vi "Main.Cleanup.vi"(11 "State Variables":T1={"Main App"={"Device Error"={"status"=FALSE, "code"=0, "source"=""}, "FPGA Session"=0, "Incoming Decimation"=0, "Outgoing Decimation"=0, "Process"=refnum}, "Protocol App"={"XNET Settings"={"Database"="", "Cluster"="", "Port"="", "Baud rate [Bd]"=0, "Termination"=0, "Incoming Rate"=0, "Outcoming Rate"=1, "Write Decimation"=1}, "Data"=[], "DTCs"=[], "Sim Addresses LUT"=variant, "Data Table LUT"=variant, "MonitorTool.Network"={"Address"=0, "Name"=0}, "Name"=""}} {"Protocol App"."MonitorTool.Network"."Name" format="%.0x"; "Protocol App"."Data"."Trigger.Refs"."Data Reference" format="%.0x"; "Protocol App"."Data"."Disable.Refs"."Data Reference" format="%.0x"; "Protocol App"."Data"."Timing.Refs"."Data Reference" format="%.0x"; "Protocol App"."Data"."Network"."Name" format="%.0x"; "Protocol App"."Data"."Incoming.Refs"."Data Reference" format="%.0x"; "Protocol App"."Data"."Outgoing.Refs"."Data Reference" format="%.0x"; "Protocol App"."XNET Settings"."Termination" items=["Off", "On"]}) -> (0 "error out":errorcluster)   [LabVIEW 2015, in "J1939 Addon Engine.lvlib"]
uses:
  J1939 Addon Engine.lvlib
  Types/Main.State Variables.ctl
  <vilib>/NI/NIVS Inline Async API/_VS Inline Async API/VS Inline Async API/VS Inline Async API.lvclass
  Types/Main.Settings.ctl
  Types/Protocol.App Settings.ctl
  Shared/Types/XNET Settings.ctl
  Types/Protocol.XNET Refs.ctl
  Shared/Types/Monitor Settings.ctl
  <vilib>/NI Veristand/Custom Device API/Block Data Reference.ctl
  <vilib>/NI Veristand/Custom Device API/Data Reference.ctl
  Types/Main.Outgoing.Frame.Settings.ctl
  Shared/Types/Outgoing Event Trigger Types.ctl
  Types/Engine.DTC Settings.ctl
  Shared/Types/Compiled Simulated Settings.ctl
  Types/Engine.DTC FIFOs.ctl
  <vilib>/xnet/xnet.llb/XNET Database Close (Database).vi
  <vilib>/NI VeriStand/Custom Device API/Custom Device API.lvlib
  Shared/J1939 Addon Shared.lvlib
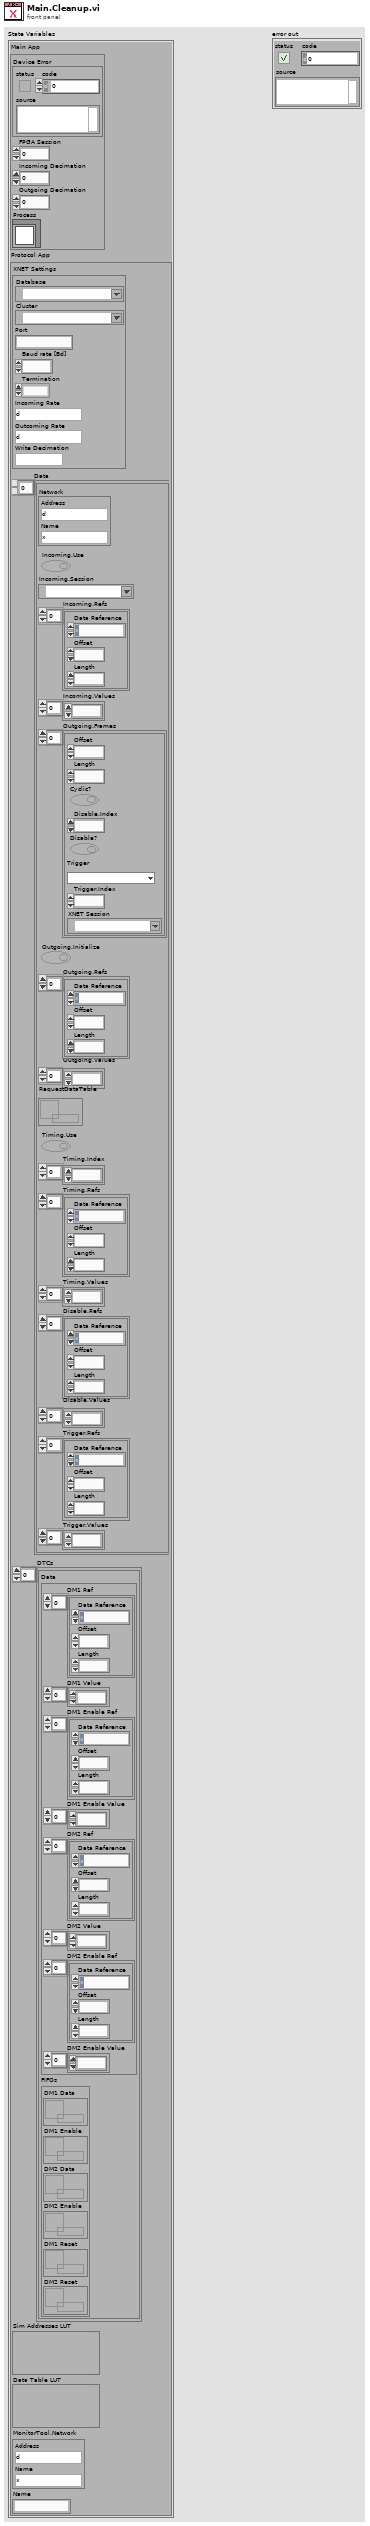
[diagram p1: front panel]
types:
  T1 = typedef "J1939 Addon Engine.lvlib/Main.State Variables.ctl" = cluster{"Main App":T2, "Protocol App":T3}
  T2 = typedef "J1939 Addon Engine.lvlib/Main.Settings.ctl" = cluster{"Device Error":errorcluster, "FPGA Session":u32, "Incoming Decimation":u32, "Outgoing Decimation":u32, "Process":refnum<class "VS Inline Async API.lvclass">}
  T3 = typedef "J1939 Addon Engine.lvlib/Protocol.App Settings.ctl" = cluster{"XNET Settings":T4, "Data":T5[], "DTCs":T11[], "Sim Addresses LUT":variant, "Data Table LUT":variant, "MonitorTool.Network":T6, "Name":string}
  T4 = typedef "J1939 Addon Shared.lvlib/XNET Settings.ctl" = cluster{"Database":refnum<k21>, "Cluster":refnum<k21>, "Port":string, "Baud rate [Bd]":u32, "Termination":u32, "Incoming Rate":u32, "Outcoming Rate":u32, "Write Decimation":u32}
  T5 = typedef "J1939 Addon Engine.lvlib/Protocol.XNET Refs.ctl" = cluster{"Network":T6, "Incoming.Use":bool, "Incoming.Session":refnum<k21>, "Incoming.Refs":T7[], "Incoming.Values":dbl[], "Outgoing.Frames":T9[], "Outgoing.Initialize":bool, "Outgoing.Refs":T7[], "Outgoing.Values":dbl[], "RequestDataTable":refnum<k33>, "Timing.Use":bool, "Timing.Index":i32[], "Timing.Refs":T7[], "Timing.Values":dbl[], "Disable.Refs":T7[], "Disable.Values":dbl[], "Trigger.Refs":T7[], "Trigger.Values":dbl[]}
  T6 = typedef "J1939 Addon Shared.lvlib/Monitor Settings.ctl" = cluster{"Address":u8, "Name":u64}
  T7 = typedef "Custom Device API.lvlib/Block Data Reference.ctl" = cluster{"Data Reference":T8, "Offset":u64, "Length":u64}
  T8 = typedef "Custom Device API.lvlib/Data Reference.ctl" = i32
  T9 = typedef "J1939 Addon Engine.lvlib/Main.Outgoing.Frame.Settings.ctl" = cluster{"Offset":u32, "Length":u32, "Cyclic?":bool, "Disable.Index":i32, "Disable?":bool, "Trigger":T10, "Trigger.Index":i32, "XNET Session":refnum<k21>}
  T10 = typedef "J1939 Addon Shared.lvlib/Outgoing Event Trigger Types.ctl" = enum16{"Channel value change", "Trigger channel (not zero)", "Channel value change or trigger channel (not zero)", "Trigger channel (any value change)", "Channel value change or trigger channel (any value change)"}
  T11 = typedef "J1939 Addon Engine.lvlib/Engine.DTC Settings.ctl" = cluster{"Data":T12, "FIFOs":T13}
  T12 = typedef "J1939 Addon Shared.lvlib/Compiled Simulated Settings.ctl" = cluster{"DM1 Ref":T7[], "DM1 Value":dbl[], "DM1 Enable Ref":T7[], "DM1 Enable Value":dbl[], "DM2 Ref":T7[], "DM2 Value":dbl[], "DM2 Enable Ref":T7[], "DM2 Enable Value":dbl[]}
  T13 = typedef "J1939 Addon Engine.lvlib/Engine.DTC FIFOs.ctl" = cluster{"DM1 Data":refnum<k33>, "DM1 Enable":refnum<k33>, "DM2 Data":refnum<k33>, "DM2 Enable":refnum<k33>, "DM1 Reset":refnum<k33>, "DM2 Reset":refnum<k33>}
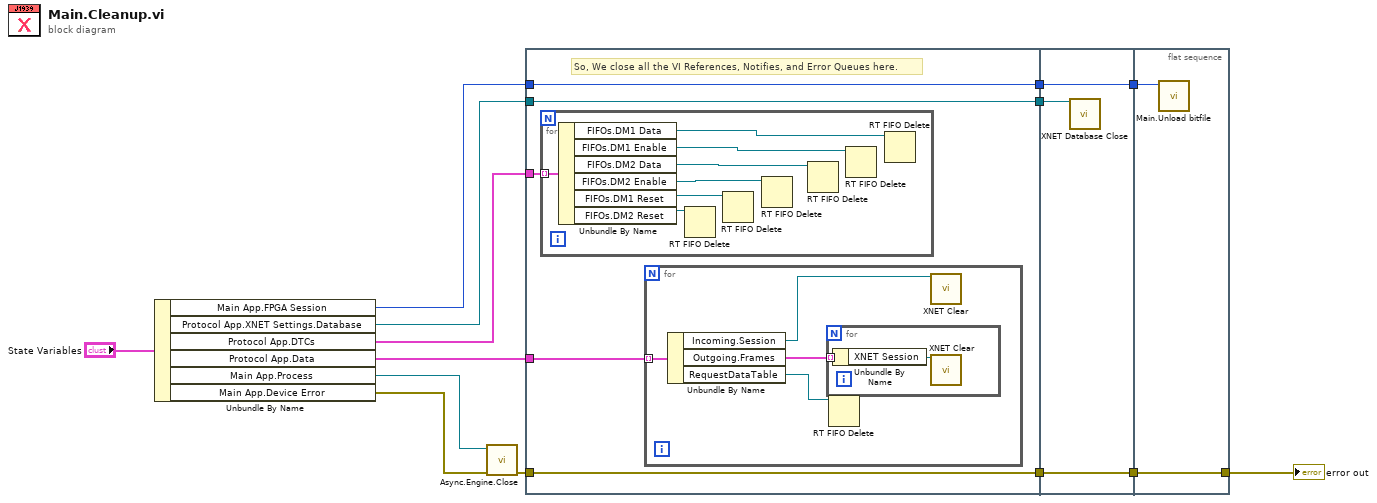
[diagram p0: block diagram]
diagram:
  n1 = Unbundle By Name("State Variables") -> ("Main App.FPGA Session"=w5:u32, "Protocol App.XNET Settings.Database"=w8:refnum<k21>, "Protocol App.DTCs"=w9:T11[], "Protocol App.Data"=w6:T5[], "Main App.Process"=w3:refnum<class "VS Inline Async API.lvclass">, "Main App.Device Error"=w2:errorcluster)
  n2 = call <vilib>:"Async.Engine.Close.vi"("error in (no error)"=w2, "Async in"=w3) -> ("error out"=w4:errorcluster)  [unwired: 8 in, 1 out]
  n3 = flat-sequence {
    tunnel: w4 -> [w19]
    tunnel: w8 -> [w18]
    tunnel: [w19] -> w14
    tunnel: [w18] -> w13
    tunnel: [w17] -> w12
    tunnel: w5 -> [w17]
    tunnel: w9 -> [w16]
    tunnel: w6 -> [w15]
    tunnel: w14 -> [w35]
    tunnel: w13 -> [w34]
    tunnel: [w35] -> w11
    tunnel: [w33] -> w10
    tunnel: w12 -> [w33]
    tunnel: [w37] -> w1
    tunnel: w11 -> [w37]
    tunnel: w10 -> [w36]
    frame #0 {
      # "So, We close all the VI References, Notifies, and Error Queues here."
      n4 = for {
        tunnel: w16 -> [w26] mode=indexing
        n5 = Unbundle By Name(w26) -> ("FIFOs.DM1 Data"=w25:refnum<k33>, "FIFOs.DM1 Enable"=w24:refnum<k33>, "FIFOs.DM2 Data"=w23:refnum<k33>, "FIFOs.DM2 Enable"=w20:refnum<k33>, "FIFOs.DM1 Reset"=w21:refnum<k33>, "FIFOs.DM2 Reset"=w22:refnum<k33>)
        n6 = RT FIFO Delete(0:w22) -> ()  [unwired: 2 in, 1 out]
        n7 = RT FIFO Delete(0:w21) -> ()  [unwired: 2 in, 1 out]
        n8 = RT FIFO Delete(0:w20) -> ()  [unwired: 2 in, 1 out]
        n9 = RT FIFO Delete(0:w23) -> ()  [unwired: 2 in, 1 out]
        n10 = RT FIFO Delete(0:w24) -> ()  [unwired: 2 in, 1 out]
        n11 = RT FIFO Delete(0:w25) -> ()  [unwired: 2 in, 1 out]
      }
      n12 = for {
        tunnel: w15 -> [w28] mode=indexing
        n13 = Unbundle By Name(w28) -> ("Incoming.Session"=w30:refnum<k21>, "Outgoing.Frames"=w29:T9[], "RequestDataTable"=w27:refnum<k33>)
        n14 = for {
          tunnel: w29 -> [w32] mode=indexing
          n15 = Unbundle By Name(w32) -> ("XNET Session"=w31:refnum<k21>)
          n16 = call <vilib>:"XNET Clear.vi"("session in"=w31) -> ()  [unwired: 14 in, 1 out]
        }
        n17 = RT FIFO Delete(0:w27) -> ()  [unwired: 2 in, 1 out]
        n18 = call <vilib>:"XNET Clear.vi"("session in"=w30) -> ()  [unwired: 14 in, 1 out]
      }
    }
    frame #1 {
      n19 = call-poly <vilib>:"XNET Database Close.vi"("database in"=w34) -> ()  [unwired: 14 in, 1 out]
    }
    frame #2 {
      n20 = call "Main.Unload bitfile.vi"("Session"=w36) -> ()  [unwired: 11 in]
    }
  }
  "error out" <- w1
